vi "Instrument Status.vi"(8 "error in (no error)":errorcluster, 11 "VISA resource name":refnum<visa-resource-name>) -> (0 "error out":errorcluster, 2 "Status Info":string, 3 "VISA resource name out":refnum<visa-resource-name>)   [LabVIEW 2017, in "ScientiFic DC Power Supply.lvlib"]
doc: "Resets the status of Instrument with Hex Format"
uses:
  ScientiFic DC Power Supply.lvlib
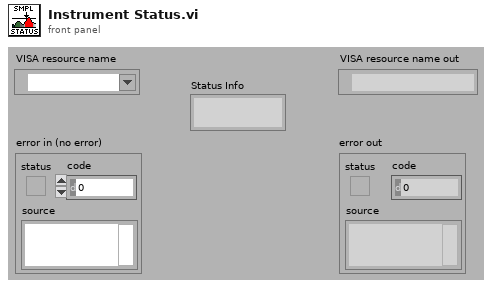
[diagram p1: front panel]
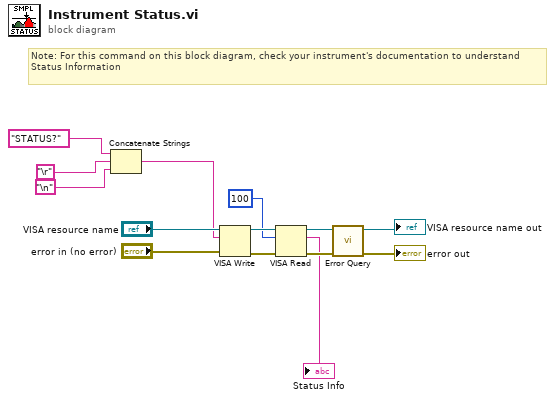
[diagram p0: block diagram]
diagram:
  # "Note: For this command on this block diagram, check your instrument's documentation to understand Status Information"
  n1 = Concatenate Strings("STATUS?" ("write buffer"), "\r", "\n") -> (w7:string)
  n2 = VISA Write(VISA resource name="VISA resource name", write buffer=w7, error in (no error)="error in (no error)") -> (VISA resource name out=w5:refnum<visa-resource-name>, error out=w6:errorcluster)  [unwired: 1 out]
  n3 = VISA Read(VISA resource name=w5, byte count=u32 100, error in (no error)=w6) -> (VISA resource name out=w4:refnum<visa-resource-name>, read buffer=→"Status Info":string, error out=w3:errorcluster)  [unwired: 1 out]
  n4 = call "Error Query.vi"("error in (no error)"=w3, "VISA resource name"=w4) -> ("error out"=→"error out":errorcluster, "VISA resource name out"=→"VISA resource name out":refnum<visa-resource-name>)  [unwired: 8 in]
